vi "scanvec_diffmethods.vi"(6 "Mode":enum16{"Vertical", "Zigzag", "Horizontal"}(ring), 8 "y pixels":dbl, 9 "x pixels":dbl, 10 "y range":dbl[](array[numeric]), 11 "x range":dbl[](array[numeric])) -> (1 "yvec":dbl[](array[numeric]), 2 "xvec":dbl[](array[numeric]))   [LabVIEW 2017]
uses:
  <vilib>/imath/engines/lvmath2/RunTimeEngine/IndexRead/NIMS V(S).vi
  <instcachedir>/0/NIMS V(S)_0488751826AF41519A22953C041130DC.lvgen/NIMS V(S)_0488751826AF41519A22953C041130DC_000.vi
  <vilib>/imath/engines/lvmath2/RunTimeEngine/BuiltInFunctions/linramp/NIMS_linramp.vi
  <vilib>/imath/engines/lvmath2/RunTimeEngine/ErrorHandling/NIMS_Create Error From Enums.vi
  <vilib>/imath/engines/lvmath2/RunTimeEngine/BuiltInFunctions/repeatmx/NIMS_repeatmx(GM, I32, I32).vi
  <instcachedir>/0/NIMS_repeatmx(GM, I32, I32)_8EDBB852F26742A48D04758F158AC943.lvgen/NIMS_repeatmx(GM, I32, I32)_8EDBB852F26742A48D04758F158AC943_000.vi
  <vilib>/imathl/engines/lvmath/Functions/Error Handling/Create Error.vi
  <vilib>/imath/engines/lvmath2/RunTimeEngine/IndexRead/NIMS M($).vi
  <instcachedir>/0/NIMS M($)_82D1177398184AFB96A6AFB63C3C3F57.lvgen/NIMS M($)_82D1177398184AFB96A6AFB63C3C3F57_000.vi
  <vilib>/imath/engines/lvmath2/RunTimeEngine/IndexRead/NIMS M($,S).vi
  <instcachedir>/0/NIMS M($,S)_3E5749BBB62E49528D4765A77F1F6D98.lvgen/NIMS M($,S)_3E5749BBB62E49528D4765A77F1F6D98_000.vi
  <vilib>/imath/engines/lvmath2/RunTimeEngine/NodeEndStatement/NIMS_NodeEndStatement_Output.vi
  <instcachedir>/0/NIMS_NodeEndStatement_Output_53EC0D466D134D7ABD903AC30B43404B.lvgen/NIMS_NodeEndStatement_Output_53EC0D466D134D7ABD903AC30B43404B_005.vi
  <vilib>/imath/engines/lvmath2/RunTimeEngine/ErrorHandling/NIMS_Finalize Error.vi
  <vilib>/imath/engines/lvmath2/RunTimeEngine/RangeToken/NIMS_Range.vi
  <instcachedir>/0/NIMS_Range_69CB9AAD882742A19CF7E739BE79952C.lvgen/NIMS_Range_69CB9AAD882742A19CF7E739BE79952C_000.vi
  <vilib>/imath/engines/lvmath2/RunTimeSupport/NIMS_Error if Not Equal.vi
  <instcachedir>/0/NIMS_Error if Not Equal_6374CBDCC5AA461FB337545605D07630.lvgen/NIMS_Error if Not Equal_6374CBDCC5AA461FB337545605D07630_001.vi
  <vilib>/imath/engines/lvmath2/RunTimeEngine/IndexRead/NIMS V(V).vi
  <instcachedir>/0/NIMS V(V)_298D9CB7BFEB42B8BC8D9C3C28AE8C70.lvgen/NIMS V(V)_298D9CB7BFEB42B8BC8D9C3C28AE8C70_000.vi
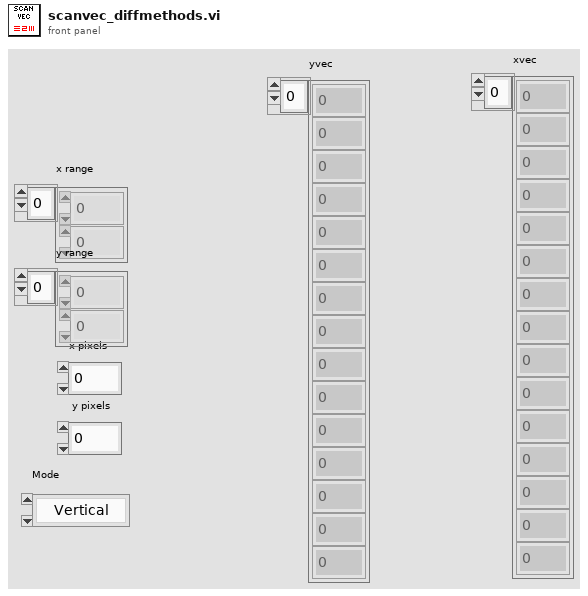
[diagram p1: front panel]
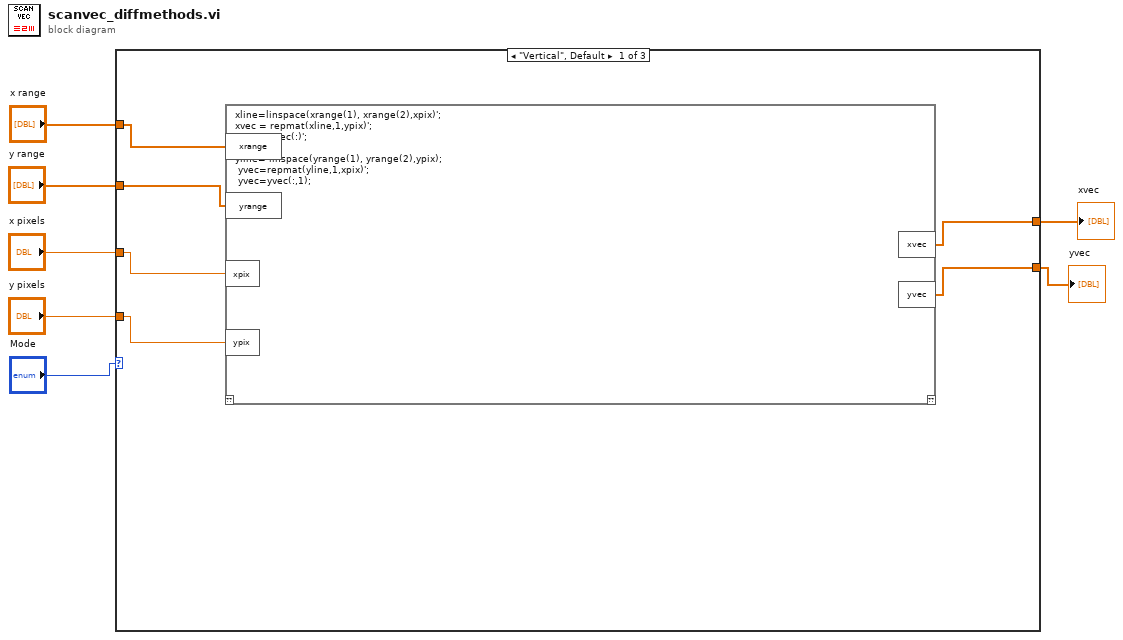
[diagram p0: block diagram]
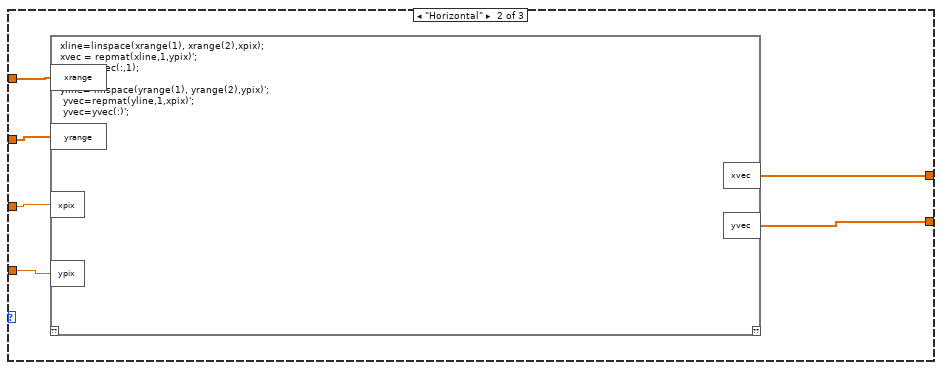
[diagram p2: hidden frame]
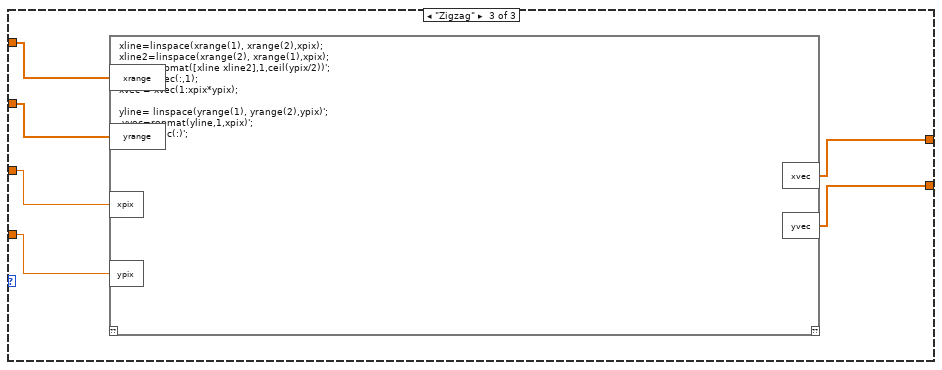
[diagram p3: hidden frame]
diagram:
  n1 = case shown="\"Vertical\", Default" "Mode" {
    tunnel: "y pixels" -> [w10 w177 w337]
    tunnel: "x pixels" -> [w11 w176 w338]
    tunnel: "y range" -> [w12 w175 w339]
    tunnel: "x range" -> [w13 w174 w340]
    tunnel: [w9 w173 w341] -> w2
    tunnel: [w8 w172 w336] -> w1
    frame "Vertical", Default {
      n2 = mathscript code="xline=linspace(xrange(1), xrange(2),xpix)';\nxvec = repmat(xline,1,ypix)';\nxvec = xvec(:)';\n\nyline= linspace(yrange(1), yrange(2),ypix);\n yvec=repmat(yline,1,xpix)';\n yvec=yvec(:,1);"("ypix"=w10, "xpix"=w11, "yrange"=w12, "xrange"=w13) -> ("xvec"=w8:dbl[], "yvec"=w9:dbl[])  [unwired: 1 in, 1 out]
    }
    frame "Horizontal" {
      n3 = mathscript code="xline=linspace(xrange(1), xrange(2),xpix);\nxvec = repmat(xline,1,ypix)';\nxvec = xvec(:,1);\n\nyline= linspace(yrange(1), yrange(2),ypix)';\n yvec=repmat(yline,1,xpix)';\n yvec=yvec(:)';"("ypix"=w177, "xpix"=w176, "yrange"=w175, "xrange"=w174) -> ("xvec"=w172:dbl[], "yvec"=w173:dbl[])  [unwired: 1 in, 1 out]
    }
    frame "Zigzag" {
      n4 = mathscript code="xline=linspace(xrange(1), xrange(2),xpix);\nxline2=linspace(xrange(2), xrange(1),xpix);\nxvec = repmat([xline xline2],1,ceil(ypix/2))';\nxvec = xvec(:,1);\nxvec = xvec(1:xpix*ypix);\n\nyline= linspace(yrange(1), yrange(2),ypix)';\n yvec=repmat(yline,1,xpix)';\n yvec=yvec(:)';"("ypix"=w337, "xpix"=w338, "yrange"=w339, "xrange"=w340) -> ("xvec"=w336:dbl[], "yvec"=w341:dbl[])  [unwired: 1 in, 1 out]
    }
  }
  "yvec" <- w2
  "xvec" <- w1
